vi "DisplayJson.vi"(11 "JSON String In":string="[{\"version\":\"1.0.0\",\"header\":{\"creationDate\":\"2022-06-03T00:00:00\",\"remarks\":\"\",\"serialNumber\":\"98172\",\"productNumber\":\"123021.1804\",\"productType\":\"PAA-9L\",\"pressureType\":2,\"productSeries\":\"9L\",\"compensatedTemperatureRange\":{\"min\":-10.0,\"max\":80.0,\"unit\":4},\"compensatedPressureRange\":{\"min\":0.0,\"max\":0.35,\"unit\":3},\"electricSupply\":{\"magnitude\":1.0,\"unit\":18},\"orderNumber\":9990266,\"orderPosition\":3,\"orderTargetDispatchDate\":\"2022-06-02T00:00:00+00:00\",\"customerName\":\"DemoData Inc.\",\"customerNumber\":12345678,\"customerOrderNumber\":\"Cust-9990266-123\",\"customerReferenceNumber\":\"\",\"customerProductT...") -> ()   [LabVIEW 2017] (continued)
\":0.349982,\"unit\":3},\"error\":{\"magnitude\":-0.0042246526,\"unit\":7}},\"temperature\":{\"output\":{\"magnitude\":80.0718,\"unit\":4},\"error\":{\"magnitude\":0.12046292,\"unit\":4}}}}}}]},{\"version\":\"1.0.0\",\"header\":{\"creationDate\":\"2022-06-03T00:00:00\",\"remarks\":\"\",\"serialNumber\":\"98131\",\"productNumber\":\"123021.1804\",\"productType\":\"PAA-9L\",\"pressureType\":2,\"productSeries\":\"9L\",\"compensatedTemperatureRange\":{\"min\":-10.0,\"max\":80.0,\"unit\":4},\"compensatedPressureRange\":{\"min\":0.0,\"max\":0.35,\"unit\":3},\"electricSupply\":{\"magnitude\":1.0,\"unit\":18},\"orderNumber\":9990266,\"orderPosition\":3,\"orderTargetDispatchDate\":\"2022-06-02T00:00:00+00:00\",\"customerName\":\"DemoData Inc.\",\"customerNumber\":12345678,\"customerOrderNumber\":\"Cust-9990266-123\",\"customerReferenceNumber\":\"\",\"customerProductType\":\"123021-1804 Rev.AA\"},\"compensationMethods\":{\"mathematicalModels\":{\"MM0123\":{\"modelType\":\"MM0123\",\"productNumber\":\"000000.0000\",\"compensatedTemperatureRange\":{\"min\":-10.0,\"max\":80.0,\"unit\":4},\"compensatedPressureRange\":{\"min\":0.0,\"max\":0.35,\"unit\":3},\"electricSupply\":{\"magnitude\":1.0,\"unit\":18},\"parts\":{\"pressure\":{\"inputs\":[\"Sig\",\"R\"],\"output\":\"P\",\"description\":\"P = f(Sig,R)\",\"coefficients\":[[4.73720301423,-0.00483633925469,1.83351336414E-06,-3.10937568343E-10,1.97386974438E-14],[-0.154436349951,0.000166317890162,-6.39343800602E-08,1.09169899896E-11,-6.99994868917E-16],[0.00010362586329,-8.07962057229E-08,2.16496396582E-11,-2.0508430231E-15,1.95096740952E-20]]},\"temperature\":{\"inputs\":[\"R\",\"Sig\"],\"output\":\"T\",\"description\":\"T = f(R,Sig)\",\"coefficients\":[[-8248.33548656,15.737062096,-0.164013492642],[8.15139219868,-0.0161407387204,0.000178198052903],[-0.00308666644108,6.23892452973E-06,-7.25606717381E-08],[5.2907699758E-07,-1.07342223159E-09,1.31183736733E-11],[-3.42100075743E-11,6.93000054124E-14,-8.89282851713E-16]]}}}}},\"measurements\":[{\"reference\":\"F_12300_XX_0000098765\",\"environmentTarget\":{\"pressure\":{\"magnitude\":0.03,\"unit\":3},\"temperature\":{\"magnitude\":-10.0,\"unit\":4}},\"environment\":{\"pressure\":{\"magnitude\":0.0300042,\"unit\":3},\"temperature\":{\"magnitude\":-10.7286,\"unit\":4},\"supply\":{\"magnitude\":1.0,\"unit\":18}},\"raw\":{\"signal\":{\"magnitude\":15.623178184,\"unit\":22},\"bridgeResistance\":{\"magnitude\":3262.5696894,\"unit\":28}},\"compensated\":{\"mathematicalModels\":{\"MM0123\":{\"pressure\":{\"output\":{\"magnitude\":0.0300109,\"unit\":3},\"error\":{\"magnitude\":0.0019239821,\"unit\":7}},\"temperature\":{\"output\":{\"magnitude\":-10.8399,\"unit\":4},\"error\":{\"magnitude\":-0.1122443,\"unit\":4}}}}}},{\"reference\":\"F_12300_XX_0000098765\",\"environmentTarget\":{\"pressure\":{\"magnitude\":0.11,\"unit\":3},\"temperature\":{\"magnitude\":-10.0,\"unit\":4}},\"environment\":{\"pressure\":{\"magnitude\":0.109992,\"unit\":3},\"temperature\":{\"magnitude\":-10.7286,\"unit\":4},\"supply\":{\"magnitude\":1.0,\"unit\":18}},\"raw\":{\"signal\":{\"magnitude\":26.228194744,\"unit\":22},\"bridgeResistance\":{\"magnitude\":3258.6192657,\"unit\":28}},\"compensated\":{\"mathematicalModels\":{\"MM0123\":{\"pressure\":{\"output\":{\"magnitude\":0.109965,\"unit\":3},\"error\":{\"magnitude\":-0.0076455132,\"unit\":7}},\"temperature\":{\"output\":{\"magnitude\":-10.8393,\"unit\":4},\"error\":{\"magnitude\":-0.11066155,\"unit\":4}}}}}},{\"reference\":\"F_12300_XX_0000098765\",\"environmentTarget\":{\"pressure\":{\"magnitude\":0.19,\"unit\":3},\"temperature\":{\"magnitude\":-10.0,\"unit\":4}},\"environment\":{\"pressure\":{\"magnitude\":0.190006,\"unit\":3},\"temperature\":{\"magnitude\":-10.7286,\"unit\":4},\"supply\":{\"magnitude\":1.0,\"unit\":18}},\"raw\":{\"signal\":{\"magnitude\":36.806694974,\"unit\":22},\"bridgeResistance\":{\"magnitude\":3254.7338558,\"unit\":28}},\"compensated\":{\"mathematicalModels\":{\"MM0123\":{\"pressure\":{\"output\":{\"magnitude\":0.190012,\"unit\":3},\"error\":{\"magnitude\":0.0018372209,\"unit\":7}},\"temperature\":{\"output\":{\"magnitude\":-10.8414,\"unit\":4},\"error\":{\"magnitude\":-0.11274271,\"unit\":4}}}}}},{\"reference\":\"F_12300_XX_0000098765\",\"environmentTarget\":{\"pressure\":{\"magnitude\":0.27,\"unit\":3},\"temperature\":{\"magnitude\":-10.0,\"unit\":4}},\"environment\":{\"pressure\":{\"magnitude\":0.270005,\"unit\":3},\"temperature\":{\"magnitude\":-10.7286,\"unit\":4},\"supply\":{\"magnitude\":1.0,\"unit\":18}},\"raw\":{\"signal\":{\"magnitude\":47.342528464,\"unit\":22},\"bridgeResistance\":{\"magnitude\":3250.9760143,\"unit\":28}},\"compensated\":{\"mathematicalModels\":{\"MM0123\":{\"pressure\":{\"output\":{\"magnitude\":0.27003,\"unit\":3},\"error\":{\"magnitude\":0.0072362262,\"unit\":7}},\"temperature\":{\"output\":{\"magnitude\":-10.838,\"unit\":4},\"error\":{\"magnitude\":-0.10936606,\"unit\":4}}}}}},{\"reference\":\"F_12300_XX_0000098765\",\"environmentTarget\":{\"pressure\":{\"magnitude\":0.35,\"unit\":3},\"temperature\":{\"magnitude\":-10.0,\"unit\":4}},\"environment\":{\"pressure\":{\"magnitude\":0.350006,\"unit\":3},\"temperature\":{\"magnitude\":-10.7286,\"unit\":4},\"supply\":{\"magnitude\":1.0,\"unit\":18}},\"raw\":{\"signal\":{\"magnitude\":57.832890395,\"unit\":22},\"bridgeResistance\":{\"magnitude\":3247.2686615,\"unit\":28}},\"compensated\":{\"mathematicalModels\":{\"MM0123\":{\"pressure\":{\"output\":{\"magnitude\":0.350002,\"unit\":3},\"error\":{\"magnitude\":-0.0010304877,\"unit\":7}},\"temperature\":{\"output\":{\"magnitude\":-10.8415,\"unit\":4},\"error\":{\"magnitude\":-0.11286831,\"unit\":4}}}}}},{\"reference\":\"F_12300_XX_0000098765\",\"environmentTarget\":{\"pressure\":{\"magnitude\":0.03,\"unit\":3},\"temperature\":{\"magnitude\":0.0,\"unit\":4}},\"environment\":{\"pressure\":{\"magnitude\":0.029999,\"unit\":3},\"temperature\":{\"magnitude\":-0.629962,\"unit\":4},\"supply\":{\"magnitude\":1.0,\"unit\":18}},\"raw\":{\"signal\":{\"magnitude\":16.089015787,\"unit\":22},\"bridgeResistance\":{\"magnitude\":3331.4612951,\"unit\":28}},\"compensated\":{\"mathematicalModels\":{\"MM0123\":{\"pressure\":{\"output\":{\"magnitude\":0.0300169,\"unit\":3},\"error\":{\"magnitude\":0.0051075138,\"unit\":7}},\"temperature\":{\"output\":{\"magnitude\":-0.741416,\"unit\":4},\"error\":{\"magnitude\":-0.11245419,\"unit\":4}}}}}},{\"reference\":\"F_12300_XX_0000098765\",\"environmentTarget\":{\"pressure\":{\"magnitude\":0.11,\"unit\":3},\"temperature\":{\"magnitude\":0.0,\"unit\":4}},\"environment\":{\"pressure\":{\"magnitude\":0.110001,\"unit\":3},\"temperature\":{\"magnitude\":-0.629962,\"unit\":4},\"supply\":{\"magnitude\":1.0,\"unit\":18}},\"raw\":{\"signal\":{\"magnitude\":26.663132376,\"unit\":22},\"bridgeResistance\":{\"magnitude\":3327.4906823,\"unit\":28}},\"compensated\":{\"mathematicalModels\":{\"MM0123\":{\"pressure\":{\"output\":{\"magnitude\":0.109982,\"unit\":3},\"error\":{\"magnitude\":-0.0055320873,\"unit\":7}},\"temperature\":{\"output\":{\"magnitude\":-0.748001,\"unit\":4},\"error\":{\"magnitude\":-0.11803924,\"unit\":4}}}}}},{\"reference\":\"F_12300_XX_0000098765\",\"environmentTarget\":{\"pressure\":{\"magnitude\":0.19,\"unit\":3},\"temperature\":{\"magnitude\":0.0,\"unit\":4}},\"environment\":{\"pressure\":{\"magnitude\":0.190003,\"unit\":3},\"temperature\":{\"magnitude\":-0.629962,\"unit\":4},\"supply\":{\"magnitude\":1.0,\"unit\":18}},\"raw\":{\"signal\":{\"magnitude\":37.209483242,\"unit\":22},\"bridgeResistance\":{\"magnitude\":3323.6474436,\"unit\":28}},\"compensated\":{\"mathematicalModels\":{\"MM0123\":{\"pressure\":{\"output\":{\"magnitude\":0.190001,\"unit\":3},\"error\":{\"magnitude\":-0.00052205368,\"unit\":7}},\"temperature\":{\"output\":{\"magnitude\":-0.746824,\"unit\":4},\"error\":{\"magnitude\":-0.11686236,\"unit\":4}}}}}},{\"reference\":\"F_12300_XX_0000098765\",\"environmentTarget\":{\"pressure\":{\"magnitude\":0.27,\"unit\":3},\"temperature\":{\"magnitude\":0.0,\"unit\":4}},\"environment\":{\"pressure\":{\"magnitude\":0.269997,\"unit\":3},\"temperature\":{\"magnitude\":-0.629962,\"unit\":4},\"supply\":{\"magnitude\":1.0,\"unit\":18}},\"raw\":{\"signal\":{\"magnitude\":47.7173752,\"unit\":22},\"bridgeResistance\":{\"magnitude\":3319.8529636,\"unit\":28}},\"compensated\":{\"mathematicalModels\":{\"MM0123\":{\"pressure\":{\"output\":{\"magnitude\":0.270007,\"unit\":3},\"error\":{\"magnitude\":0.0029559519,\"unit\":7}},\"temperature\":{\"output\":{\"magnitude\":-0.749689,\"unit\":4},\"error\":{\"magnitude\":-0.11972714,\"unit\":4}}}}}},{\"reference\":\"F_12300_XX_0000098765\",\"environmentTarget\":{\"pressure\":{\"magnitude\":0.35,\"unit\":3},\"temperature\":{\"magnitude\":0.0,\"unit\":4}},\"environment\":{\"pressure\":{\"magnitude\":0.350001,\"unit\":3},\"temperature\":{\"magnitude\":-0.629962,\"unit\":4},\"supply\":{\"magnitude\":1.0,\"unit\":18}},\"raw\":{\"signal\":{\"magnitude\":58.183891314,\"unit\":22},\"bridgeResistance\":{\"magnitude\":3316.1332902,\"unit\":28}},\"compensated\":{\"mathematicalModels\":{\"MM0123\":{\"pressure\":{\"output\":{\"magnitude\":0.349978,\"unit\":3},\"error\":{\"magnitude\":-0.0066521209,\"unit\":7}},\"temperature\":{\"output\":{\"magnitude\":-0.753319,\"unit\":4},\"error\":{\"magnitude\":-0.12335746,\"unit\":4}}}}}},{\"reference\":\"F_12300_XX_0000098765\",\"environmentTarget\":{\"pressure\":{\"magnitude\":0.03,\"unit\":3},\"temperature\":{\"magnitude\":20.0,\"unit\":4}},\"environment\":{\"pressure\":{\"magnitude\":0.0299929,\"unit\":3},\"temperature\":{\"magnitude\":19.5509,\"unit\":4},\"supply\":{\"magnitude\":1.0,\"unit\":18}},\"raw\":{\"signal\":{\"magnitude\":17.05096908,\"unit\":22},\"bridgeResistance\":{\"magnitude\":3486.4220046,\"unit\":28}},\"compensated\":{\"mathematicalModels\":{\"MM0123\":{\"pressure\":{\"output\":{\"magnitude\":0.0299956,\"unit\":3},\"error\":{\"magnitude\":0.00076416833,\"unit\":7}},\"temperature\":{\"output\":{\"magnitude\":19.5436,\"unit\":4},\"error\":{\"magnitude\":-0.0073127198,\"unit\":4}}}}}},{\"reference\":\"F_12300_XX_0000098765\",\"environmentTarget\":{\"pressure\":{\"magnitude\":0.11,\"unit\":3},\"temperature\":{\"magnitude\":20.0,\"unit\":4}},\"environment\":{\"pressure\":{\"magnitude\":0.110005,\"unit\":3},\"temperature\":{\"magnitude\":19.5509,\"unit\":4},\"supply\":{\"magnitude\":1.0,\"unit\":18}},\"raw\":{\"signal\":{\"magnitude\":27.618759294,\"unit\":22},\"bridgeResistance\":{\"magnitude\":3482.4740763,\"unit\":28}},\"compensated\":{\"mathematicalModels\":{\"MM0123\":{\"pressure\":{\"output\":{\"magnitude\":0.10998,\"unit\":3},\"error\":{\"magnitude\":-0.0072283987,\"unit\":7}},\"temperature\":{\"output\":{\"magnitude\":19.5407,\"unit\":4},\"error\":{\"magnitude\":-0.01019127,\"unit\":4}}}}}},{\"reference\":\"F_12300_XX_0000098765\",\"environmentTarget\":{\"pressure\":{\"magnitude\":0.19,\"unit\":3},\"temperature\":{\"magnitude\":20.0,\"unit\":4}},\"environment\":{\"pressure\":{\"magnitude\":0.190002,\"unit\":3},\"temperature\":{\"magnitude\":19.5509,\"unit\":4},\"supply\":{\"magnitude\":1.0,\"unit\":18}},\"raw\":{\"signal\":{\"magnitude\":38.160441003,\"unit\":22},\"bridgeResistance\":{\"magnitude\":3478.6075818,\"unit\":28}},\"compensated\":{\"mathematicalModels\":{\"MM0123\":{\"pressure\":{\"output\":{\"magnitude\":0.19001,\"unit\":3},\"error\":{\"magnitude\":0.0023553572,\"unit\":7}},\"temperature\":{\"output\":{\"magnitude\":19.5396,\"unit\":4},\"error\":{\"magnitude\":-0.01126324,\"unit\":4}}}}}},{\"reference\":\"F_12300_XX_0000098765\",\"environmentTarget\":{\"pressure\":{\"magnitude\":0.27,\"unit\":3},\"temperature\":{\"magnitude\":20.0,\"unit\":4}},\"environment\":{\"pressure\":{\"magnitude\":0.269994,\"unit\":3},\"temperature\":{\"magnitude\":19.5509,\"unit\":4},\"supply\":{\"magnitude\":1.0,\"unit\":18}},\"raw\":{\"signal\":{\"magnitude\":48.666968903,\"unit\":22},\"bridgeResistance\":{\"magnitude\":3474.7790758,\"unit\":28}},\"compensated\":{\"mathematicalModels\":{\"MM0123\":{\"pressure\":{\"output\":{\"magnitude\":0.270021,\"unit\":3},\"error\":{\"magnitude\":0.0077567796,\"unit\":7}},\"temperature\":{\"output\":{\"magnitude\":19.5346,\"unit\":4},\"error\":{\"magnitude\":-0.016230905,\"unit\":4}}}}}},{\"reference\":\"F_12300_XX_0000098765\",\"environmentTarget\":{\"pressure\":{\"magnitude\":0.35,\"unit\":3},\"temperature\":{\"magnitude\":20.0,\"unit\":4}},\"environment\":{\"pressure\":{\"magnitude\":0.350009,\"unit\":3},\"temperature\":{\"magnitude\":19.5509,\"unit\":4},\"supply\":{\"magnitude\":1.0,\"unit\":18}},\"raw\":{\"signal\":{\"magnitude\":59.138726089,\"unit\":22},\"bridgeResistance\":{\"magnitude\":3471.0414298,\"unit\":28}},\"compensated\":{\"mathematicalModels\":{\"MM0123\":{\"pressure\":{\"output\":{\"magnitude\":0.350013,\"unit\":3},\"error\":{\"magnitude\":0.0010844278,\"unit\":7}},\"temperature\":{\"output\":{\"magnitude\":19.5323,\"unit\":4},\"error\":{\"magnitude\":-0.018616559,\"unit\":4}}}}}},{\"reference\":\"F_12300_XX_0000098765\",\"environmentTarget\":{\"pressure\":{\"magnitude\":0.03,\"unit\":3},\"temperature\":{\"magnitude\":40.0,\"unit\":4}},\"environment\":{\"pressure\":{\"magnitude\":0.0299959,\"unit\":3},\"temperature\":{\"magnitude\":39.7284,\"unit\":4},\"supply\":{\"magnitude\":1.0,\"unit\":18}},\"raw\":{\"signal\":{\"magnitude\":18.089043385,\"unit\":22},\"bridgeResistance\":{\"magnitude\":3661.2528668,\"unit\":28}},\"compensated\":{\"mathematicalModels\":{\"MM0123\":{\"pressure\":{\"output\":{\"magnitude\":0.0300112,\"unit\":3},\"error\":{\"magnitude\":0.0043570561,\"unit\":7}},\"temperature\":{\"output\":{\"magnitude\":39.7224,\"unit\":4},\"error\":{\"magnitude\":-0.0059901864,\"unit\":4}}}}}},{\"reference\":\"F_12300_XX_0000098765\",\"environmentTarget\":{\"pressure\":{\"magnitude\":0.11,\"unit\":3},\"temperature\":{\"magnitude\":40.0,\"unit\":4}},\"environment\":{\"pressure\":{\"magnitude\":0.110002,\"unit\":3},\"temperature\":{\"magnitude\":39.7284,\"unit\":4},\"supply\":{\"magnitude\":1.0,\"unit\":18}},\"raw\":{\"signal\":{\"magnitude\":28.702628661,\"unit\":22},\"bridgeResistance\":{\"magnitude\":3657.2854047,\"unit\":28}},\"compensated\":{\"mathematicalModels\":{\"MM0123\":{\"pressure\":{\"output\":{\"magnitude\":0.109985,\"unit\":3},\"error\":{\"magnitude\":-0.0047668929,\"unit\":7}},\"temperature\":{\"output\":{\"magnitude\":39.7231,\"unit\":4},\"error\":{\"magnitude\":-0.0053208722,\"unit\":4}}}}}},{\"reference\":\"F_12300_XX_0000098765\",\"environmentTarget\":{\"pressure\":{\"magnitude\":0.19,\"unit\":3},\"temperature\":{\"magnitude\":40.0,\"unit\":4}},\"environment\":{\"pressure\":{\"magnitude\":0.190007,\"unit\":3},\"temperature\":{\"magnitude\":39.7284,\"unit\":4},\"supply\":{\"magnitude\":1.0,\"unit\":18}},\"raw\":{\"signal\":{\"magnitude\":39.293491676,\"unit\":22},\"bridgeResistance\":{\"magnitude\":3653.3301025,\"unit\":28}},\"compensated\":{\"mathematicalModels\":{\"MM0123\":{\"pressure\":{\"output\":{\"magnitude\":0.190002,\"unit\":3},\"error\":{\"magnitude\":-0.0015007021,\"unit\":7}},\"temperature\":{\"output\":{\"magnitude\":39.7177,\"unit\":4},\"error\":{\"magnitude\":-0.010739705,\"unit\":4}}}}}},{\"reference\":\"F_12300_XX_0000098765\",\"environmentTarget\":{\"pressure\":{\"magnitude\":0.27,\"unit\":3},\"temperature\":{\"magnitude\":40.0,\"unit\":4}},\"environment\":{\"pressure\":{\"magnitude\":0.269998,\"unit\":3},\"temperature\":{\"magnitude\":39.7284,\"unit\":4},\"supply\":{\"magnitude\":1.0,\"unit\":18}},\"raw\":{\"signal\":{\"magnitude\":49.855029422,\"unit\":22},\"bridgeResistance\":{\"magnitude\":3649.5038707,\"unit\":28}},\"compensated\":{\"mathematicalModels\":{\"MM0123\":{\"pressure\":{\"output\":{\"magnitude\":0.270012,\"unit\":3},\"error\":{\"magnitude\":0.0041172249,\"unit\":7}},\"temperature\":{\"output\":{\"magnitude\":39.7187,\"unit\":4},\"error\":{\"magnitude\":-0.0096879162,\"unit\":4}}}}}},{\"reference\":\"F_12300_XX_0000098765\",\"environmentTarget\":{\"pressure\":{\"magnitude\":0.35,\"unit\":3},\"temperature\":{\"magnitude\":40.0,\"unit\":4}},\"environment\":{\"pressure\":{\"magnitude\":0.350006,\"unit\":3},\"temperature\":{\"magnitude\":39.7284,\"unit\":4},\"supply\":{\"magnitude\":1.0,\"unit\":18}},\"raw\":{\"signal\":{\"magnitude\":60.382712563,\"unit\":22},\"bridgeResistance\":{\"magnitude\":3645.7287332,\"unit\":28}},\"compensated\":{\"mathematicalModels\":{\"MM0123\":{\"pressure\":{\"output\":{\"magnitude\":0.349986,\"unit\":3},\"error\":{\"magnitude\":-0.0055763284,\"unit\":7}},\"temperature\":{\"output\":{\"magnitude\":39.7175,\"unit\":4},\"error\":{\"magnitude\":-0.010896761,\"unit\":4}}}}}},{\"reference\":\"F_12300_XX_0000098765\",\"environmentTarget\":{\"pressure\":{\"magnitude\":0.03,\"unit\":3},\"temperature\":{\"magnitude\":60.0,\"unit\":4}},\"environment\":{\"pressure\":{\"magnitude\":0.0299999,\"unit\":3},\"temperature\":{\"magnitude\":59.8651,\"unit\":4},\"supply\":{\"magnitude\":1.0,\"unit\":18}},\"raw\":{\"signal\":{\"magnitude\":19.234311093,\"unit\":22},\"bridgeResistance\":{\"magnitude\":3852.8932957,\"unit\":28}},\"compensated\":{\"mathematicalModels\":{\"MM0123\":{\"pressure\":{\"output\":{\"magnitude\":0.0300096,\"unit\":3},\"error\":{\"magnitude\":0.0027638749,\"unit\":7}},\"temperature\":{\"output\":{\"magnitude\":59.9284,\"unit\":4},\"error\":{\"magnitude\":0.063290941,\"unit\":4}}}}}},{\"reference\":\"F_12300_XX_0000098765\",\"environmentTarget\":{\"pressure\":{\"magnitude\":0.11,\"unit\":3},\"temperature\":{\"magnitude\":60.0,\"unit\":4}},\"environment\":{\"pressure\":{\"magnitude\":0.109999,\"unit\":3},\"temperature\":{\"magnitude\":59.8651,\"unit\":4},\"supply\":{\"magnitude\":1.0,\"unit\":18}},\"raw\":{\"signal\":{\"magnitude\":29.932221802,\"unit\":22},\"bridgeResistance\":{\"magnitude\":3848.8748579,\"unit\":28}},\"compensated\":{\"mathematicalModels\":{\"MM0123\":{\"pressure\":{\"output\":{\"magnitude\":0.109976,\"unit\":3},\"error\":{\"magnitude\":-0.006487395,\"unit\":7}},\"temperature\":{\"output\":{\"magnitude\":59.9305,\"unit\":4},\"error\":{\"magnitude\":0.065327613,\"unit\":4}}}}}},{\"reference\":\"F_12300_XX_0000098765\",\"environmentTarget\":{\"pressure\":{\"magnitude\":0.19,\"unit\":3},\"temperature\":{\"magnitude\":60.0,\"unit\":4}},\"environment\":{\"pressure\":{\"magnitude\":0.190002,\"unit\":3},\"temperature\":{\"magnitude\":59.8651,\"unit\":4},\"supply\":{\"magnitude\":1.0,\"unit\":18}},\"raw\":{\"signal\":{\"magnitude\":40.612435105,\"unit\":22},\"bridgeResistance\":{\"magnitude\":3844.9225126,\"unit\":28}},\"compensated\":{\"mathematicalModels\":{\"MM0123\":{\"pressure\":{\"output\":{\"magnitude\":0.190002,\"unit\":3},\"error\":{\"magnitude\":5.0156521E-06,\"unit\":7}},\"temperature\":{\"output\":{\"magnitude\":59.933,\"unit\":4},\"error\":{\"magnitude\":0.067832162,\"unit\":4}}}}}},{\"reference\":\"F_12300_XX_0000098765\",\"environmentTarget\":{\"pressure\":{\"magnitude\":0.27,\"unit\":3},\"temperature\":{\"magnitude\":60.0,\"unit\":4}},\"environment\":{\"pressure\":{\"magnitude\":0.270007,\"unit\":3},\"temperature\":{\"magnitude\":59.8651,\"unit\":4},\"supply\":{\"magnitude\":1.0,\"unit\":18}},\"raw\":{\"signal\":{\"magnitude\":51.267442642,\"unit\":22},\"bridgeResistance\":{\"magnitude\":3840.9924393,\"unit\":28}},\"compensated\":{\"mathematicalModels\":{\"MM0123\":{\"pressure\":{\"output\":{\"magnitude\":0.270033,\"unit\":3},\"error\":{\"magnitude\":0.0074192501,\"unit\":7}},\"temperature\":{\"output\":{\"magnitude\":59.9321,\"unit\":4},\"error\":{\"magnitude\":0.06696606,\"unit\":4}}}}}},{\"reference\":\"F_12300_XX_0000098765\",\"environmentTarget\":{\"pressure\":{\"magnitude\":0.35,\"unit\":3},\"temperature\":{\"magnitude\":60.0,\"unit\":4}},\"environment\":{\"pressure\":{\"magnitude\":0.349996,\"unit\":3},\"temperature\":{\"magnitude\":59.8651,\"unit\":4},\"supply\":{\"magnitude\":1.0,\"unit\":18}},\"raw\":{\"signal\":{\"magnitude\":61.897073556,\"unit\":22},\"bridgeResistance\":{\"magnitude\":3837.1684191,\"unit\":28}},\"compensated\":{\"mathematicalModels\":{\"MM0123\":{\"pressure\":{\"output\":{\"magnitude\":0.349989,\"unit\":3},\"error\":{\"magnitude\":-0.0022534769,\"unit\":7}},\"temperature\":{\"output\":{\"magnitude\":59.9359,\"unit\":4},\"error\":{\"magnitude\":0.070744589,\"unit\":4}}}}}},{\"reference\":\"F_12300_XX_0000098765\",\"environmentTarget\":{\"pressure\":{\"magnitude\":0.03,\"unit\":3},\"temperature\":{\"magnitude\":80.0,\"unit\":4}},\"environment\":{\"pressure\":{\"magnitude\":0.0299974,\"unit\":3},\"temperature\":{\"magnitude\":79.9513,\"unit\":4},\"supply\":{\"magnitude\":1.0,\"unit\":18}},\"raw\":{\"signal\":{\"magnitude\":20.536238518,\"unit\":22},\"bridgeResistance\":{\"magnitude\":4058.9085966,\"unit\":28}},\"compensated\":{\"mathematicalModels\":{\"MM0123\":{\"pressure\":{\"output\":{\"magnitude\":0.0300103,\"unit\":3},\"error\":{\"magnitude\":0.0036714968,\"unit\":7}},\"temperature\":{\"output\":{\"magnitude\":80.049,\"unit\":4},\"error\":{\"magnitude\":0.097644655,\"unit\":4}}}}}},{\"reference\":\"F_12300_XX_0000098765\",\"environmentTarget\":{\"pressure\":{\"magnitude\":0.11,\"unit\":3},\"temperature\":{\"magnitude\":80.0,\"unit\":4}},\"environment\":{\"pressure\":{\"magnitude\":0.109999,\"unit\":3},\"temperature\":{\"magnitude\":79.9513,\"unit\":4},\"supply\":{\"magnitude\":1.0,\"unit\":18}},\"raw\":{\"signal\":{\"magnitude\":31.341798213,\"unit\":22},\"bridgeResistance\":{\"magnitude\":4054.8317304,\"unit\":28}},\"compensated\":{\"mathematicalModels\":{\"MM0123\":{\"pressure\":{\"output\":{\"magnitude\":0.109966,\"unit\":3},\"error\":{\"magnitude\":-0.00940281,\"unit\":7}},\"temperature\":{\"output\":{\"magnitude\":80.0525,\"unit\":4},\"error\":{\"magnitude\":0.10114155,\"unit\":4}}}}}},{\"reference\":\"F_12300_XX_0000098765\",\"environmentTarget\":{\"pressure\":{\"magnitude\":0.19,\"unit\":3},\"temperature\":{\"magnitude\":80.0,\"unit\":4}},\"environment\":{\"pressure\":{\"magnitude\":0.189992,\"unit\":3},\"temperature\":{\"magnitude\":79.9513,\"unit\":4},\"supply\":{\"magnitude\":1.0,\"unit\":18}},\"raw\":{\"signal\":{\"magnitude\":42.137059449,\"unit\":22},\"bridgeResistance\":{\"magnitude\":4050.8333969,\"unit\":28}},\"compensated\":{\"mathematicalModels\":{\"MM0123\":{\"pressure\":{\"output\":{\"magnitude\":0.189999,\"unit\":3},\"error\":{\"magnitude\":0.0020530745,\"unit\":7}},\"temperature\":{\"output\":{\"magnitude\":80.0592,\"unit\":4},\"error\":{\"magnitude\":0.10786722,\"unit\":4}}}}}},{\"reference\":\"F_12300_XX_0000098765\",\"environmentTarget\":{\"pressure\":{\"magnitude\":0.27,\"unit\":3},\"temperature\":{\"magnitude\":80.0,\"unit\":4}},\"environment\":{\"pressure\":{\"magnitude\":0.270004,\"unit\":3},\"temperature\":{\"magnitude\":79.9513,\"unit\":4},\"supply\":{\"magnitude\":1.0,\"unit\":18}},\"raw\":{\"signal\":{\"magnitude\":52.910203739,\"unit\":22},\"bridgeResistance\":{\"magnitude\":4046.8582164,\"unit\":28}},\"compensated\":{\"mathematicalModels\":{\"MM0123\":{\"pressure\":{\"output\":{\"magnitude\":0.270027,\"unit\":3},\"error\":{\"magnitude\":0.0065329474,\"unit\":7}},\"temperature\":{\"output\":{\"magnitude\":80.0638,\"unit\":4},\"error\":{\"magnitude\":0.11242673,\"unit\":4}}}}}},{\"reference\":\"F_12300_XX_0000098765\",\"environmentTarget\":{\"pressure\":{\"magnitude\":0.35,\"unit\":3},\"temperature\":{\"magnitude\":80.0,\"unit\":4}},\"environment\":{\"pressure\":{\"magnitude\":0.349999,\"unit\":3},\"temperature\":{\"magnitude\":79.9513,\"unit\":4},\"supply\":{\"magnitude\":1.0,\"unit\":18}},\"raw\":{\"signal\":{\"magnitude\":63.652909459,\"unit\":22},\"bridgeResistance\":{\"magnitude\":4042.9413801,\"unit\":28}},\"compensated\":{\"mathematicalModels\":{\"MM0123\":{\"pressure\":{\"output\":{\"magnitude\":0.349987,\"unit\":3},\"error\":{\"magnitude\":-0.003526305,\"unit\":7}},\"temperature\":{\"output\":{\"magnitude\":80.0693,\"unit\":4},\"error\":{\"magnitude\":0.11795127,\"unit\":4}}}}}}]},{\"version\":\"1.0.0\",\"header\":{\"creationDate\":\"2022-06-03T00:00:00\",\"remarks\":\"\",\"serialNumber\":\"98130\",\"productNumber\":\"123021.1804\",\"productType\":\"PAA-9L\",\"pressureType\":2,\"productSeries\":\"9L\",\"compensatedTemperatureRange\":{\"min\":-10.0,\"max\":80.0,\"unit\":4},\"compensatedPressureRange\":{\"min\":0.0,\"max\":0.35,\"unit\":3},\"electricSupply\":{\"magnitude\":1.0,\"unit\":18},\"orderNumber\":9990266,\"orderPosition\":3,\"orderTargetDispatchDate\":\"2022-06-02T00:00:00+00:00\",\"customerName\":\"DemoData Inc.\",\"customerNumber\":12345678,\"customerOrderNumber\":\"Cust-9990266-123\",\"customerReferenceNumber\":\"\",\"customerProductType\":\"123021-1804 Rev.AA\"},\"compensationMethods\":{\"mathematicalModels\":{\"MM0123\":{\"modelType\":\"MM0123\",\"productNumber\":\"000000.0000\",\"compensatedTemperatureRange\":{\"min\":-10.0,\"max\":80.0,\"unit\":4},\"compensatedPressureRange\":{\"min\":0.0,\"max\":0.35,\"unit\":3},\"electricSupply\":{\"magnitude\":1.0,\"unit\":18},\"parts\":{\"pressure\":{\"inputs\":[\"Sig\",\"R\"],\"output\":\"P\",\"description\":\"P = f(Sig,R)\",\"coefficients\":[[4.47893066729,-0.00455806996131,1.71987405549E-06,-2.90398015622E-10,1.83565249487E-14],[-0.143383876112,0.000154163236398,-5.89004438475E-08,9.99755754065E-12,-6.37431218455E-16],[-0.000209490732779,2.5681293948E-07,-1.14462318258E-10,2.22774862329E-14,-1.60751564503E-18]]},\"temperature\":{\"inputs\":[\"R\",\"Sig\"],\"output\":\"T\",\"description\":\"T = f(R,Sig)\",\"coefficients\":[[-8315.29190809,15.0518576012,-0.153363597104],[8.19438696464,-0.0151636109452,0.000163817306707],[-0.00309368329298,5.74961658573E-06,-6.55734913872E-08],[5.28620790262E-07,-9.69019642079E-10,1.16530530136E-11],[-3.40717339903E-11,6.11851401102E-14,-7.7555432891E-16]]}}}}},\"measurements\":[{\"reference\":\"F_12300_XX_0000098765\",\"environmentTarget\":{\"pressure\":{\"magnitude\":0.03,\"unit\":3},\"temperature\":{\"magnitude\":-10.0,\"unit\":4}},\"environment\":{\"pressure\":{\"magnitude\":0.0300042,\"unit\":3},\"temperature\":{\"magnitude\":-10.7286,\"unit\":4},\"supply\":{\"magnitude\":1.0,\"unit\":18}},\"raw\":{\"signal\":{\"magnitude\":15.851273284,\"unit\":22},\"bridgeResistance\":{\"magnitude\":3272.4857691,\"unit\":28}},\"compensated\":{\"mathematicalModels\":{\"MM0123\":{\"pressure\":{\"output\":{\"magnitude\":0.0300101,\"unit\":3},\"error\":{\"magnitude\":0.0016778453,\"unit\":7}},\"temperature\":{\"output\":{\"magnitude\":-10.8353,\"unit\":4},\"error\":{\"magnitude\":-0.10670693,\"unit\":4}}}}}},{\"reference\":\"F_12300_XX_0000098765\",\"environmentTarget\":{\"pressure\":{\"magnitude\":0.11,\"unit\":3},\"temperature\":{\"magnitude\":-10.0,\"unit\":4}},\"environment\":{\"pressure\":{\"magnitude\":0.109994,\"unit\":3},\"temperature\":{\"magnitude\":-10.7286,\"unit\":4},\"supply\":{\"magnitude\":1.0,\"unit\":18}},\"raw\":{\"signal\":{\"magnitude\":26.256252412,\"unit\":22},\"bridgeResistance\":{\"magnitude\":3268.5701455,\"unit\":28}},\"compensated\":{\"mathematicalModels\":{\"MM0123\":{\"pressure\":{\"output\":{\"magnitude\":0.109971,\"unit\":3},\"error\":{\"magnitude\":-0.0066748458,\"unit\":7}},\"temperature\":{\"output\":{\"magnitude\":-10.8348,\"unit\":4},\"error\":{\"magnitude\":-0.10620516,\"unit\":4}}}}}},{\"reference\":\"F_12300_XX_0000098765\",\"environmentTarget\":{\"pressure\":{\"magnitude\":0.19,\"unit\":3},\"temperature\":{\"magnitude\":-10.0,\"unit\":4}},\"environment\":{\"pressure\":{\"magnitude\":0.190005,\"unit\":3},\"temperature\":{\"magnitude\":-10.7286,\"unit\":4},\"supply\":{\"magnitude\":1.0,\"unit\":18}},\"raw\":{\"signal\":{\"magnitude\":36.634236148,\"unit\":22},\"bridgeResistance\":{\"magnitude\":3264.7205428,\"unit\":28}},\"compensated\":{\"mathematicalModels\":{\"MM0123\":{\"pressure\":{\"output\":{\"magnitude\":0.190013,\"unit\":3},\"error\":{\"magnitude\":0.0022604992,\"unit\":7}},\"temperature\":{\"output\":{\"magnitude\":-10.8377,\"unit\":4},\"error\":{\"magnitude\":-0.10909509,\"unit\":4}}}}}},{\"reference\":\"F_12300_XX_0000098765\",\"environmentTarget\":{\"pressure\":{\"magnitude\":0.27,\"unit\":3},\"temperature\":{\"magnitude\":-10.0,\"unit\":4}},\"environment\":{\"pressure\":{\"magnitude\":0.270006,\"unit\":3},\"temperature\":{\"magnitude\":-10.7286,\"unit\":4},\"supply\":{\"magnitude\":1.0,\"unit\":18}},\"raw\":{\"signal\":{\"magnitude\":46.970900455,\"unit\":22},\"bridgeResistance\":{\"magnitude\":3261.0241974,\"unit\":28}},\"compensated\":{\"mathematicalModels\":{\"MM0123\":{\"pressure\":{\"output\":{\"magnitude\":0.270024,\"unit\":3},\"error\":{\"magnitude\":0.0052734594,\"unit\":7}},\"temperature\":{\"output\":{\"magnitude\":-10.8322,\"unit\":4},\"error\":{\"magnitude\":-0.10352704,\"unit\":4}}}}}},{\"reference\":\"F_12300_XX_0000098765\",\"environmentTarget\":{\"pressure\":{\"magnitude\":0.35,\"unit\":3},\"temperature\":{\"magnitude\":-10.0,\"unit\":4}},\"environment\":{\"pressure\":{\"magnitude\":0.350006,\"unit\":3},\"temperature\":{\"magnitude\":-10.7286,\"unit\":4},\"supply\":{\"magnitude\":1.0,\"unit\":18}},\"raw\":{\"signal\":{\"magnitude\":57.265129758,\"unit\":22},\"bridgeResistance\":{\"magnitude\":3257.365646,\"unit\":28}},\"compensated\":{\"mathematicalModels\":{\"MM0123\":{\"pressure\":{\"output\":{\"magnitude\":0.350002,\"unit\":3},\"error\":{\"magnitude\":-0.0011574167,\"unit\":7}},\"temperature\":{\"output\":{\"magnitude\":-10.8363,\"unit\":4},\"error\":{\"magnitude\":-0.10767097,\"unit\":4}}}}}},{\"reference\":\"F_12300_XX_0000098765\",\"environmentTarget\":{\"pressure\":{\"magnitude\":0.03,\"unit\":3},\"temperature\":{\"magnitude\":0.0,\"unit\":4}},\"environment\":{\"pressure\":{\"magnitude\":0.0300043,\"unit\":3},\"temperature\":{\"magnitude\":-0.629962,\"unit\":4},\"supply\":{\"magnitude\":1.0,\"unit\":18}},\"raw\":{\"signal\":{\"magnitude\":16.294535813,\"unit\":22},\"bridgeResistance\":{\"magnitude\":3341.4167932,\"unit\":28}},\"compensated\":{\"mathematicalModels\":{\"MM0123\":{\"pressure\":{\"output\":{\"magnitude\":0.03002,\"unit\":3},\"error\":{\"magnitude\":0.0044940162,\"unit\":7}},\"temperature\":{\"output\":{\"magnitude\":-0.73978,\"unit\":4},\"error\":{\"magnitude\":-0.1098184,\"unit\":4}}}}}},{\"reference\":\"F_12300_XX_0000098765\",\"environmentTarget\":{\"pressure\":{\"magnitude\":0.11,\"unit\":3},\"temperature\":{\"magnitude\":0.0,\"unit\":4}},\"environment\":{\"pressure\":{\"magnitude\":0.110004,\"unit\":3},\"temperature\":{\"magnitude\":-0.629962,\"unit\":4},\"supply\":{\"magnitude\":1.0,\"unit\":18}},\"raw\":{\"signal\":{\"magnitude\":26.669630926,\"unit\":22},\"bridgeResistance\":{\"magnitude\":3337.5040391,\"unit\":28}},\"compensated\":{\"mathematicalModels\":{\"MM0123\":{\"pressure\":{\"output\":{\"magnitude\":0.109984,\"unit\":3},\"error\":{\"magnitude\":-0.0057247825,\"unit\":7}},\"temperature\":{\"output\":{\"magnitude\":-0.744276,\"unit\":4},\"error\":{\"magnitude\":-0.11431385,\"unit\":4}}}}}},{\"reference\":\"F_12300_XX_0000098765\",\"environmentTarget\":{\"pressure\":{\"magnitude\":0.19,\"unit\":3},\"temperature\":{\"magnitude\":0.0,\"unit\":4}},\"environment\":{\"pressure\":{\"magnitude\":0.190005,\"unit\":3},\"temperature\":{\"magnitude\":-0.629962,\"unit\":4},\"supply\":{\"magnitude\":1.0,\"unit\":18}},\"raw\":{\"signal\":{\"magnitude\":37.016773738,\"unit\":22},\"bridgeResistance\":{\"magnitude\":3333.6989777,\"unit\":28}},\"compensated\":{\"mathematicalModels\":{\"MM0123\":{\"pressure\":{\"output\":{\"magnitude\":0.190007,\"unit\":3},\"error\":{\"magnitude\":0.00048320176,\"unit\":7}},\"temperature\":{\"output\":{\"magnitude\":-0.743969,\"unit\":4},\"error\":{\"magnitude\":-0.11400722,\"unit\":4}}}}}},{\"reference\":\"F_12300_XX_0000098765\",\"environmentTarget\":{\"pressure\":{\"magnitude\":0.27,\"unit\":3},\"temperature\":{\"magnitude\":0.0,\"unit\":4}},\"environment\":{\"pressure\":{\"magnitude\":0.269998,\"unit\":3},\"temperature\":{\"magnitude\":-0.629962,\"unit\":4},\"supply\":{\"magnitude\":1.0,\"unit\":18}},\"raw\":{\"signal\":{\"magnitude\":47.324992907,\"unit\":22},\"bridgeResistance\":{\"magnitude\":3329.9529891,\"unit\":28}},\"compensated\":{\"mathematicalModels\":{\"MM0123\":{\"pressure\":{\"output\":{\"magnitude\":0.270007,\"unit\":3},\"error\":{\"magnitude\":0.0024828449,\"unit\":7}},\"temperature\":{\"output\":{\"magnitude\":-0.746553,\"unit\":4},\"error\":{\"magnitude\":-0.11659095,\"unit\":4}}}}}},{\"reference\":\"F_12300_XX_0000098765\",\"environmentTarget\":{\"pressure\":{\"magnitude\":0.35,\"unit\":3},\"temperature\":{\"magnitude\":0.0,\"unit\":4}},\"environment\":{\"pressure\":{\"magnitude\":0.350001,\"unit\":3},\"temperature\":{\"magnitude\":-0.629962,\"unit\":4},\"supply\":{\"magnitude\":1.0,\"unit\":18}},\"raw\":{\"signal\":{\"magnitude\":57.594418013,\"unit\":22},\"bridgeResistance\":{\"magnitude\":3326.279393,\"unit\":28}},\"compensated\":{\"mathematicalModels\":{\"MM0123\":{\"pressure\":{\"output\":{\"magnitude\":0.349985,\"unit\":3},\"error\":{\"magnitude\":-0.0046480942,\"unit\":7}},\"temperature\":{\"output\":{\"magnitude\":-0.750518,\"unit\":4},\"error\":{\"magnitude\":-0.12055578,\"unit\":4}}}}}},{\"reference\":\"F_12300_XX_0000098765\",\"environmentTarget\":{\"pressure\":{\"magnitude\":0.03,\"unit\":3},\"temperature\":{\"magnitude\":20.0,\"unit\":4}},\"environment\":{\"pressure\":{\"magnitude\":0.029996,\"unit\":3},\"temperature\":{\"magnitude\":19.5509,\"unit\":4},\"supply\":{\"magnitude\":1.0,\"unit\":18}},\"raw\":{\"signal\":{\"magnitude\":17.215949918,\"unit\":22},\"bridgeResistance\":{\"magnitude\":3496.5471872,\"unit\":28}},\"compensated\":{\"mathematicalModels\":{\"MM0123\":{\"pressure\":{\"output\":{\"magnitude\":0.0299996,\"unit\":3},\"error\":{\"magnitude\":0.0010258958,\"unit\":7}},\"temperature\":{\"output\":{\"magnitude\":19.5457,\"unit\":4},\"error\":{\"magnitude\":-0.0051552207,\"unit\":4}}}}}},{\"reference\":\"F_12300_XX_0000098765\",\"environmentTarget\":{\"pressure\":{\"magnitude\":0.11,\"unit\":3},\"temperature\":{\"magnitude\":20.0,\"unit\":4}},\"environment\":{\"pressure\":{\"magnitude\":0.109999,\"unit\":3},\"temperature\":{\"magnitude\":19.5509,\"unit\":4},\"supply\":{\"magnitude\":1.0,\"unit\":18}},\"raw\":{\"signal\":{\"magnitude\":27.582490969,\"unit\":22},\"bridgeResistance\":{\"magnitude\":3492.6484751,\"unit\":28}},\"compensated\":{\"mathematicalModels\":{\"MM0123\":{\"pressure\":{\"output\":{\"magnitude\":0.109977,\"unit\":3},\"error\":{\"magnitude\":-0.0062695976,\"unit\":7}},\"temperature\":{\"output\":{\"magnitude\":19.5423,\"unit\":4},\"error\":{\"magnitude\":-0.0086217701,\"unit\":4}}}}}},{\"reference\":\"F_12300_XX_0000098765\",\"environmentTarget\":{\"pressure\":{\"magnitude\":0.19,\"unit\":3},\"temperature\":{\"magnitude\":20.0,\"unit\":4}},\"environment\":{\"pressure\":{\"magnitude\":0.190001,\"unit\":3},\"temperature\":{\"magnitude\":19.5509,\"unit\":4},\"supply\":{\"magnitude\":1.0,\"unit\":18}},\"raw\":{\"signal\":{\"magnitude\":37.923893031,\"unit\":22},\"bridgeResistance\":{\"magnitude\":3489.8239728,\"unit\":28}},\"compensated\":{\"mathematicalModels\":{\"MM0123\":{\"pressure\":{\"output\":{\"magnitude\":0.190007,\"unit\":3},\"error\":{\"magnitude\":0.0017136961,\"unit\":7}},\"temperature\":{\"output\":{\"magnitude\":19.5403,\"unit\":4},\"error\":{\"magnitude\":-0.010575864,\"unit\":4}}}}}},{\"reference\":\"F_12300_XX_0000098765\",\"environmentTarget\":{\"pressure\":{\"magnitude\":0.27,\"unit\":3},\"temperature\":{\"magnitude\":20.0,\"unit\":4}},\"environment\":{\"pressure\":{\"magnitude\":0.269992,\"unit\":3},\"temperature\":{\"magnitude\":19.5509,\"unit\":4},\"supply\":{\"magnitude\":1.0,\"unit\":18}},\"raw\":{\"signal\":{\"magnitude\":48.230389578,\"unit\":22},\"bridgeResistance\":{\"magnitude\":3485.04803,\"unit\":28}},\"compensated\":{\"mathematicalModels\":{\"MM0123\":{\"pressure\":{\"output\":{\"magnitude\":0.270016,\"unit\":3},\"error\":{\"magnitude\":0.0067661602,\"unit\":7}},\"temperature\":{\"output\":{\"magnitude\":19.5363,\"unit\":4},\"error\":{\"magnitude\":-0.014607313,\"unit\":4}}}}}},{\"reference\":\"F_12300_XX_0000098765\",\"environmentTarget\":{\"pressure\":{\"magnitude\":0.35,\"unit\":3},\"temperature\":{\"magnitude\":20.0,\"unit\":4}},\"environment\":{\"pressure\":{\"magnitude\":0.350008,\"unit\":3},\"temperature\":{\"magnitude\":19.5509,\"unit\":4},\"supply\":{\"magnitude\":1.0,\"unit\":18}},\"raw\":{\"signal\":{\"magnitude\":58.502663679,\"unit\":22},\"bridgeResistance\":{\"magnitude\":3481.3543756,\"unit\":28}},\"compensated\":{\"mathematicalModels\":{\"MM0123\":{\"pressure\":{\"output\":{\"magnitude\":0.350007,\"unit\":3},\"error\":{\"magnitude\":-0.00031855645,\"unit\":7}},\"temperature\":{\"output\":{\"magnitude\":19.5343,\"unit\":4},\"error\":{\"magnitude\":-0.016596426,\"unit\":4}}}}}},{\"reference\":\"F_12300_XX_0000098765\",\"environmentTarget\":{\"pressure\":{\"magnitude\":0.03,\"unit\":3},\"temperature\":{\"magnitude\":40.0,\"unit\":4}},\"environment\":{\"pressure\":{\"magnitude\":0.0300034,\"unit\":3},\"temperature\":{\"magnitude\":39.7284,\"unit\":4},\"supply\":{\"magnitude\":1.0,\"unit\":18}},\"raw\":{\"signal\":{\"magnitude\":18.211525071,\"unit\":22},\"bridgeResistance\":{\"magnitude\":3671.577233,\"unit\":28}},\"compensated\":{\"mathematicalModels\":{\"MM0123\":{\"pressure\":{\"output\":{\"magnitude\":0.0300163,\"unit\":3},\"error\":{\"magnitude\":0.0036901465,\"unit\":7}},\"temperature\":{\"output\":{\"magnitude\":39.7212,\"unit\":4},\"error\":{\"magnitude\":-0.0072063801,\"unit\":4}}}}}},{\"reference\":\"F_12300_XX_0000098765\",\"environmentTarget\":{\"pressure\":{\"magnitude\":0.11,\"unit\":3},\"temperature\":{\"magnitude\":40.0,\"unit\":4}},\"environment\":{\"pressure\":{\"magnitude\":0.110003,\"unit\":3},\"temperature\":{\"magnitude\":39.7284,\"unit\":4},\"supply\":{\"magnitude\":1.0,\"unit\":18}},\"raw\":{\"signal\":{\"magnitude\":28.622981445,\"unit\":22},\"bridgeResistance\":{\"magnitude\":3667.6642312,\"unit\":28}},\"compensated\":{\"mathematicalModels\":{\"MM0123\":{\"pressure\":{\"output\":{\"magnitude\":0.109987,\"unit\":3},\"error\":{\"magnitude\":-0.0045945407,\"unit\":7}},\"temperature\":{\"output\":{\"magnitude\":39.7219,\"unit\":4},\"error\":{\"magnitude\":-0.0064957004,\"unit\":4}}}}}},{\"reference\":\"F_12300_XX_0000098765\",\"environmentTarget\":{\"pressure\":{\"magnitude\":0.19,\"unit\":3},\"temperature\":{\"magnitude\":40.0,\"unit\":4}},\"environment\":{\"pressure\":{\"magnitude\":0.190009,\"unit\":3},\"temperature\":{\"magnitude\":39.7284,\"unit\":4},\"supply\":{\"magnitude\":1.0,\"unit\":18}},\"raw\":{\"signal\":{\"magnitude\":39.012243277,\"unit\":22},\"bridgeResistance\":{\"magnitude\":3663.7756192,\"unit\":28}},\"compensated\":{\"mathematicalModels\":{\"MM0123\":{\"pressure\":{\"output\":{\"magnitude\":0.190006,\"unit\":3},\"error\":{\"magnitude\":-0.00089894974,\"unit\":7}},\"temperature\":{\"output\":{\"magnitude\":39.7183,\"unit\":4},\"error\":{\"magnitude\":-0.010077381,\"unit\":4}}}}}},{\"reference\":\"F_12300_XX_0000098765\",\"environmentTarget\":{\"pressure\":{\"magnitude\":0.27,\"unit\":3},\"temperature\":{\"magnitude\":40.0,\"unit\":4}},\"environment\":{\"pressure\":{\"magnitude\":0.269995,\"unit\":3},\"temperature\":{\"magnitude\":39.7284,\"unit\":4},\"supply\":{\"magnitude\":1.0,\"unit\":18}},\"raw\":{\"signal\":{\"magnitude\":49.371308402,\"unit\":22},\"bridgeResistance\":{\"magnitude\":3659.9757899,\"unit\":28}},\"compensated\":{\"mathematicalModels\":{\"MM0123\":{\"pressure\":{\"output\":{\"magnitude\":0.270009,\"unit\":3},\"error\":{\"magnitude\":0.0039355749,\"unit\":7}},\"temperature\":{\"output\":{\"magnitude\":39.7172,\"unit\":4},\"error\":{\"magnitude\":-0.011222345,\"unit\":4}}}}}},{\"reference\":\"F_12300_XX_0000098765\",\"environmentTarget\":{\"pressure\":{\"magnitude\":0.35,\"unit\":3},\"temperature\":{\"magnitude\":40.0,\"unit\":4}},\"environment\":{\"pressure\":{\"magnitude\":0.349996,\"unit\":3},\"temperature\":{\"magnitude\":39.7284,\"unit\":4},\"supply\":{\"magnitude\":1.0,\"unit\":18}},\"raw\":{\"signal\":{\"magnitude\":59.698357579,\"unit\":22},\"bridgeResistance\":{\"magnitude\":3656.2485486,\"unit\":28}},\"compensated\":{\"mathematicalModels\":{\"MM0123\":{\"pressure\":{\"output\":{\"magnitude\":0.349982
